vi "Main.vi"() -> ()   [LabVIEW 2017]
doc: "The myRIO Project template acquires acceleration data from the onboard accelerometer and displays the changes of acceleration values in a waveform chart."
uses:
  Motor Status Enum.ctl
  Encoder Cluster.ctl
  <vilib>/myRIO/Common/Instrument Driver Framework/myRIO v1.0/Encoder/typedefs/Encoder Count Direction Enum.ctl
  Motion Type Def.ctl
  XY Cluster.ctl
  <vilib>/myRIO/Instrument Drivers/Onboard IO/PWM/typedefs/PWM Reference.ctl
  <vilib>/myRIO/Common/Instrument Driver Framework/Utilities/typedefs/myRIO Generic Hardware Reference.ctl
  <vilib>/myRIO/Common/Instrument Driver Framework/Utilities/typedefs/Hardware Version Enum.ctl
  <vilib>/myRIO/Common/Instrument Driver Framework/Utilities/typedefs/myRIO v1.0 Reference.ctl
  <vilib>/myRIO/Common/Instrument Driver Framework/Utilities/typedefs/Generic FPGA Reference.ctl
  <vilib>/myRIO/Common/Instrument Driver Framework/myRIO v1.0/PWM/typedefs/PWM Channels Enum.ctl
  <vilib>/myRIO/Instrument Drivers/Onboard IO/PWM/typedefs/PWM Configuration.ctl
  <vilib>/userdefined/High Color/nirio_resource_hc.ctl
  <vilib>/myRIO/Common/Instrument Driver Framework/Utilities/vis/Is FPGA Ref Available.vi
  <vilib>/myRIO/Common/Instrument Driver Framework/myRIO v1.0/PWM/vis/myRIO v1.1 Open PWM.vi
  <vilib>/myRIO/Instrument Drivers/Onboard IO/PWM/vis/Set Duty Cycle and Frequency.vi
  <vilib>/myRIO/Common/Instrument Driver Framework/Utilities/vis/Validate Channels.vi
  <vilib>/myRIO/Common/Instrument Driver Framework/myRIO v1.0/PWM/vis/myRIO v1.0 Reserve PWM.vi
  <vilib>/myRIO/Common/Instrument Driver Framework/myRIO v1.0/UART/vis/myRIO v1.0 Close UART.vi
  <vilib>/myRIO/Common/Instrument Driver Framework/myRIO v1.0/PWM/vis/myRIO v1.0 Build MUX Configuration PWM.vi
  <vilib>/myRIO/Common/Instrument Driver Framework/myRIO v1.0/Resource Manager/vis/myRIO v1.0 Reserve Channel List.vi
  <vilib>/myRIO/Common/Instrument Driver Framework/myRIO v1.0/Resource Manager/vis/myRIO v1.0 Create Configuration List.vi
  <vilib>/myRIO/Common/Instrument Driver Framework/myRIO v1.0/Resource Manager/vis/myRIO v1.0 Reserve Channel.vi
  <vilib>/myRIO/Common/Instrument Driver Framework/myRIO v1.0/Resource Manager/vis/myRIO v1.0 Unreserve Channel.vi
  <vilib>/myRIO/Common/Instrument Driver Framework/myRIO v1.0/Resource Manager/vis/myRIO v1.0 Build Mutex Name.vi
  <vilib>/addons/control/pid/pid.llb/PID Control Input Filter (DBL).vi
  <vilib>/addons/control/pid/pid.llb/PID (DBL).vi
  <vilib>/Utility/VariantDataType/GetNumericInfo.vi
  <vilib>/Utility/error.llb/Error Cluster From Error Code.vi
  <vilib>/myRIO/Common/Instrument Driver Framework/myRIO v1.0/myRIO v1.1 Open.vi
  <vilib>/myRIO/Common/Instrument Driver Framework/Utilities/vis/IO Manager.vi
  <vilib>/myRIO/Common/Instrument Driver Framework/Utilities/vis/Configuration Manager.vi
  <vilib>/myRIO/Common/Instrument Driver Framework/myRIO v1.0/Resource Manager/vis/myRIO v1.0 Configure IO.vi
  <vilib>/myRIO/Common/Instrument Driver Framework/myRIO v1.0/myRIO v1.0 Close.vi
  <vilib>/myRIO/Common/Instrument Driver Framework/myRIO v1.0/PWM/vis/myRIO v1.0 Write PWM.vi
  <vilib>/myRIO/Common/Instrument Driver Framework/Utilities/vis/FPGA Ref Manager.vi
  <vilib>/myRIO/Common/Instrument Driver Framework/myRIO v1.0/myRIO v1.0 Reset FPGA.vi
  <vilib>/myRIO/Common/Instrument Driver Framework/myRIO v1.0/IRQ/vis/myRIO v1.0 IRQ Info FGV.vi
  <vilib>/myRIO/Common/Instrument Driver Framework/myRIO v1.0/IRQ/vis/myRIO v1.0 Timer IRQ Info FGV.vi
  <vilib>/myRIO/Common/Instrument Driver Framework/myRIO v1.0/IRQ/vis/myRIO v1.0 ISR Agent.vi
  <vilib>/myRIO/Express VI/Onboard IO/PWM/PWM Express VI.xnode
  <vilib>/myRIO/Instrument Drivers/Onboard IO/PWM/vis/myRIO PWM Open.xnode
  <vilib>/myRIO/Instrument Drivers/Utilities/Utilities.lvlib
  <vilib>/myRIO/Instrument Drivers/Onboard IO/PWM/PWM.lvlib
  <vilib>/addons/control/pid/NI_PID_pid.lvlib
  <vilib>/ptbypt/NI_PtbyPt.lvlib
panel:
  in  "Y Input":T1
  in  "Y Axis PID":cluster{"Kc":dbl, "Ti":dbl, "Td":dbl}
  in  "X Input":T1
  in  "X Axis PID":cluster{"Kc":dbl, "Ti":dbl, "Td":dbl}
  out "Y dist > +20":bool
  out "X dist > +20":bool
  out "Y Data.Path. Profile":T2=enum."Triangular"
  out "X Data.Path.Profile":T2=enum."Triangular"
  out "Timing":T3
  out "Y PID":cluster{"Speed":dbl, "Speed":dbl}(graph)
  out "X PID":cluster{"Speed":dbl, "Speed":dbl}(graph)
  out "Encoder Output":T4
  out "Y Data.State":T6
  out "X Data.State":T6
  in  "stop":bool
  out "X&Y Complete":bool
  out "Y Displacement":dbl[](graph)
  out "X Displacement":dbl[](graph)
  out "Y Velocity":cluster{"V actual":dbl[]}[](graph)
  out "X Velocity":cluster{"V actual":dbl[]}[](graph)
  out "Y Data.Motion":T7
  out "X Data.Motion":T7
  out "Y Data.Motor Params":T8
  out "X Data.Motor Params":T9
  # "X MaxV = 26.73 mm/s at 50 Hz"
  # "Y MaxV = 14.38 mm/s at 3200 µSteps/rev"
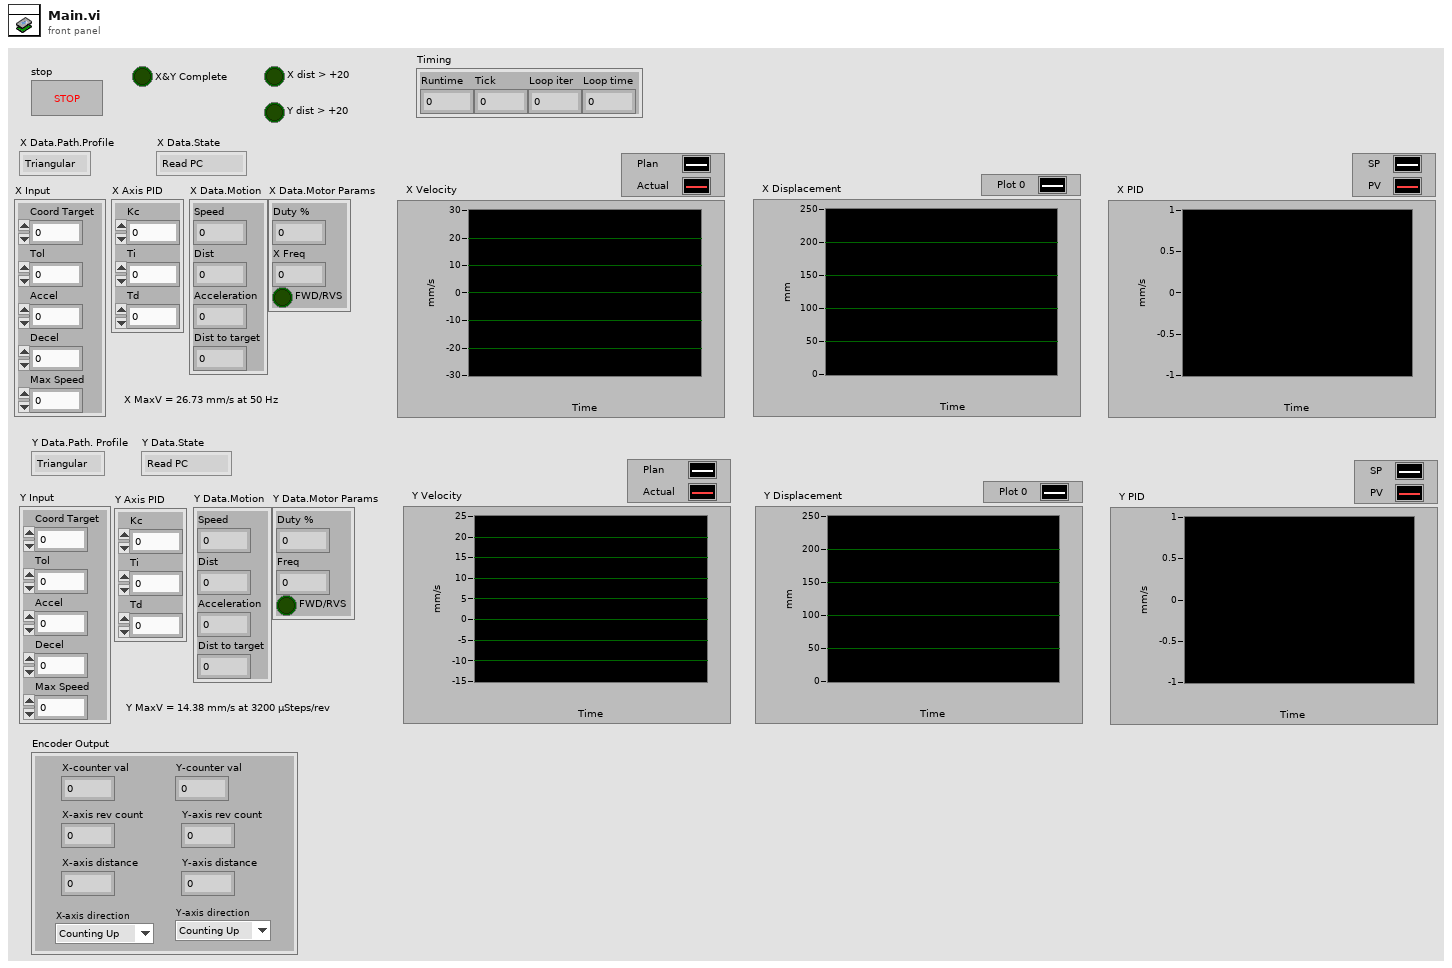
[diagram p1: front panel]
types:
  T1 = cluster{"Coord Target":dbl, "Tol":dbl, "Accel":dbl, "Decel":dbl, "Max Speed":dbl}
  T2 = typedef "Motion Type Def.ctl" = enum16{"Trapezodial", "Triangular"}
  T3 = cluster{"Runtime":dbl, "Loop time":dbl, "Loop iter":i32, "Tick":dbl}
  T4 = typedef "Encoder Cluster.ctl" = cluster{"Y-axis rev count":dbl, "Y-axis distance":dbl, "X-axis rev count":dbl, "X-axis distance":dbl, "Y-axis direction":T5, "X-axis direction":T5, "X-counter val":i32, "Y-counter val":i32}
  T5 = typedef "Encoder Count Direction Enum.ctl" = enum16{"Counting Up", "Counting Down"}
  T6 = typedef "Motor Status Enum.ctl" = enum16{"Read PC", "Stop", "Move"}
  T7 = cluster{"Speed":dbl, "Dist":dbl, "Acceleration":dbl, "Dist to target":dbl}
  T8 = cluster{"Duty %":dbl, "Freq":dbl, "FWD/RVS":bool}
  T9 = cluster{"Duty %":dbl, "X Freq":dbl, "FWD/RVS":bool}
  T10 = typedef "XY Cluster.ctl" = cluster{"X Data":cluster{"Complete?":bool, "Motor Params":cluster{"Duty %":dbl, "X Freq":dbl, "FWD/RVS":bool}, "State":T6, "Input":cluster{"Coord Target":dbl, "Tol":dbl, "Accel":dbl, "Decel":dbl, "Max Speed":dbl}, "Path":cluster{"Speed plan":dbl[], "Profile":T2, "Max Speed":dbl}, "PID":cluster{"Kc":dbl, "Ti":dbl, "Td":dbl}, "Motion":cluster{"Speed":dbl, "Dist":dbl, "Accel":dbl, "Dist Remain":dbl}, "Time step i":i32}, "Y Data":cluster{"Complete?":bool, "Motor Params":cluster{"Duty %":dbl, "Freq":dbl, "FWD/RVS":bool}, "State":T6, "Path":cluster{"Speed plan":dbl[], " Profile":T2, "Max Speed":dbl}, "PID":cluster{"Kc":dbl, "Ti":dbl, "Td":dbl}, "Motion":cluster{"Speed":dbl, "Dist":dbl, "Accel":dbl, "Dist Remain":dbl}, "Input":cluster{"Coord Target":dbl, "Tol":dbl, "Accel":dbl, "Decel":dbl, "Max Speed":dbl}, "Time step i":i32}, "Timing":cluster{"Runtime":dbl, "Loop time":dbl, "Loop iter":i32, "Tick":dbl}, "stop":bool}
  T11 = cluster{"Dist to target (mm)":dbl, "Max Speed (mm/s)":dbl, "Max Accel (mm/s^2)":dbl, "Max Decel (mm/s^2)":dbl, "Step Time (s)":dbl}
  T12 = cluster{"Complete?":bool, "Motor Params":cluster{"Duty %":dbl, "X Freq":dbl, "FWD/RVS":bool}, "State":T6, "Input":cluster{"Coord Target":dbl, "Tol":dbl, "Accel":dbl, "Decel":dbl, "Max Speed":dbl}, "Path":cluster{"Speed plan":dbl[], "Profile":T2, "Max Speed":dbl}, "PID":cluster{"Kc":dbl, "Ti":dbl, "Td":dbl}, "Motion":cluster{"Speed":dbl, "Dist":dbl, "Accel":dbl, "Dist Remain":dbl}, "Time step i":i32}
  T13 = cluster{"Coord Target":bool, "Tol":bool, "Accel":bool, "Decel":bool, "Max Speed":bool}
  T14 = cluster{"Complete?":bool, "Motor Params":cluster{"Duty %":dbl, "Freq":dbl, "FWD/RVS":bool}, "State":T6, "Path":cluster{"Speed plan":dbl[], " Profile":T2, "Max Speed":dbl}, "PID":cluster{"Kc":dbl, "Ti":dbl, "Td":dbl}, "Motion":cluster{"Speed":dbl, "Dist":dbl, "Accel":dbl, "Dist Remain":dbl}, "Input":cluster{"Coord Target":dbl, "Tol":dbl, "Accel":dbl, "Decel":dbl, "Max Speed":dbl}, "Time step i":i32}
  T15 = cluster{"Speed":dbl, "Dist":dbl, "Accel":dbl, "Dist Remain":dbl}
  T16 = cluster{"Runtime":dbl, "Dist":dbl, "Speed":dbl, "Accel":dbl, "Dist":dbl, "Speed":dbl, "Accel":dbl}
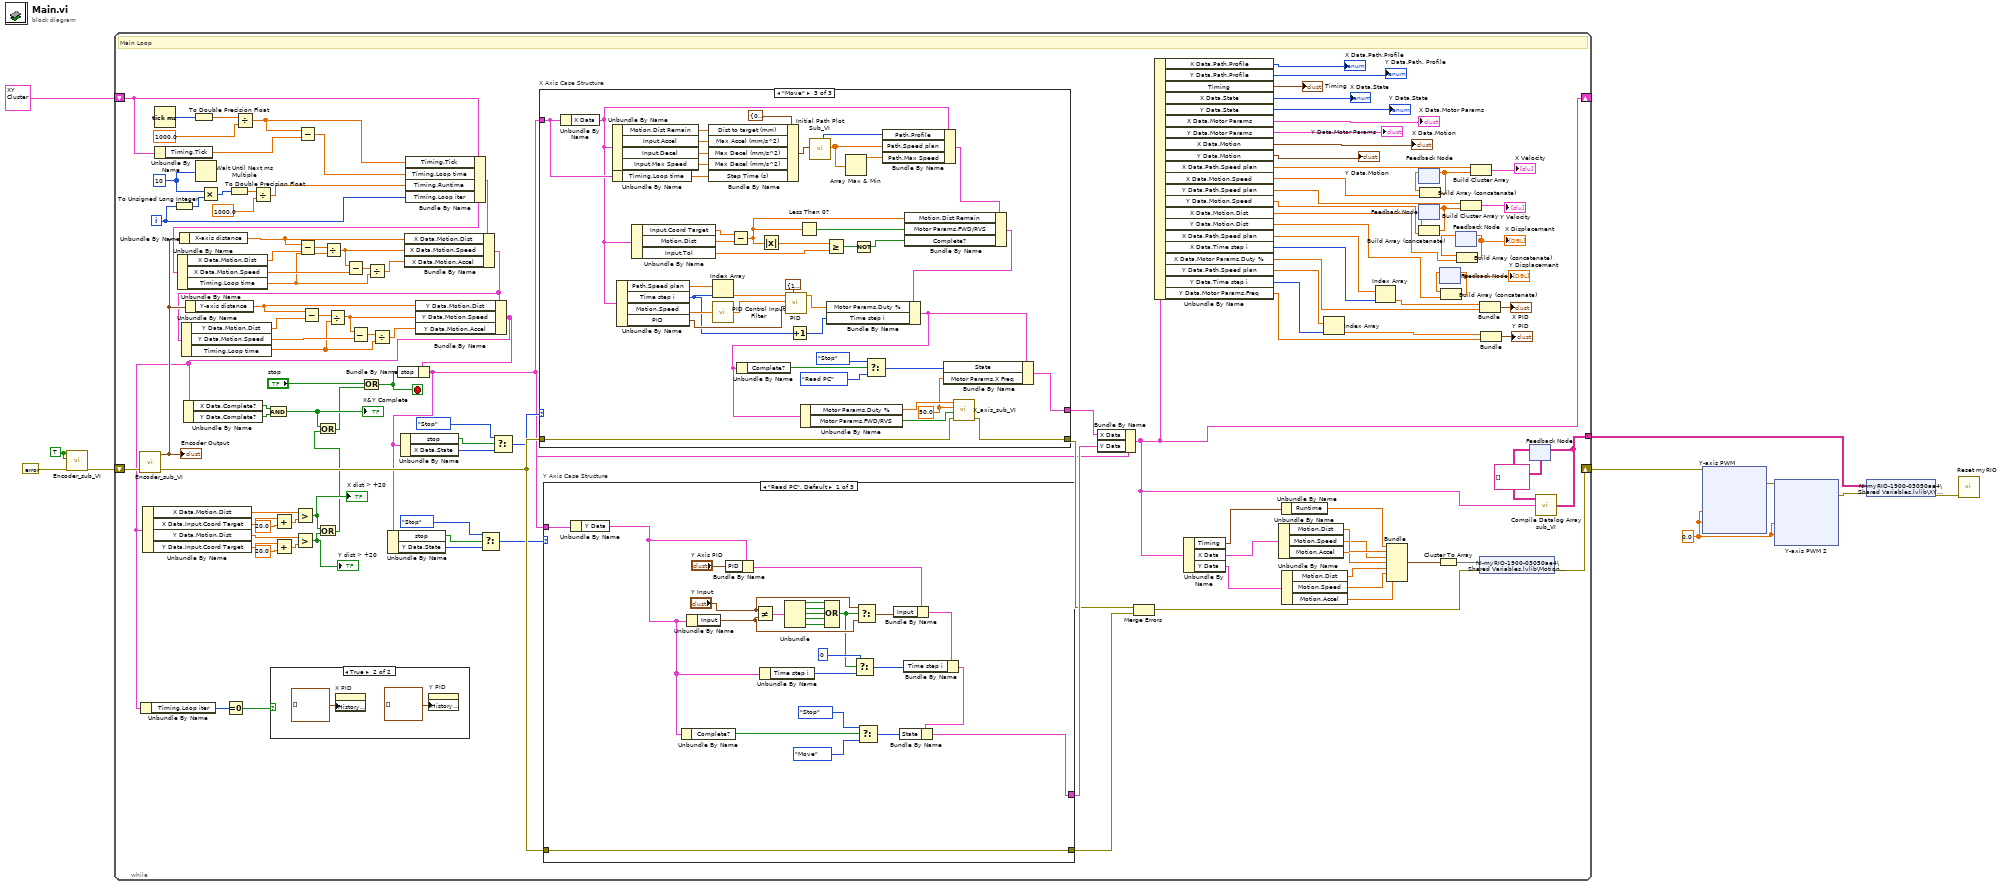
[diagram p0: block diagram]
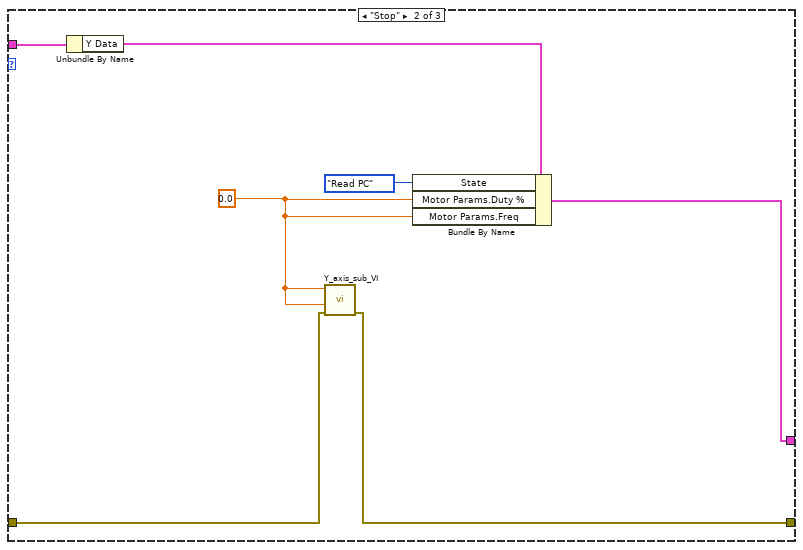
[diagram p3: hidden frame]
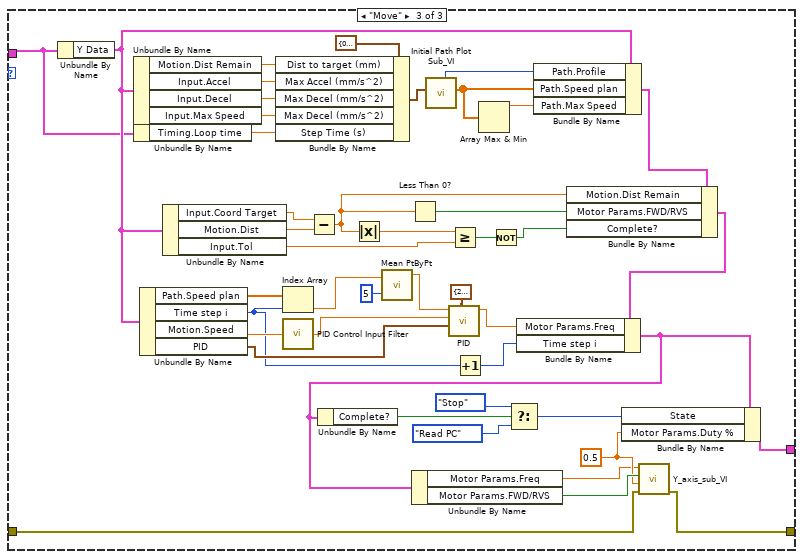
[diagram p4: hidden frame]
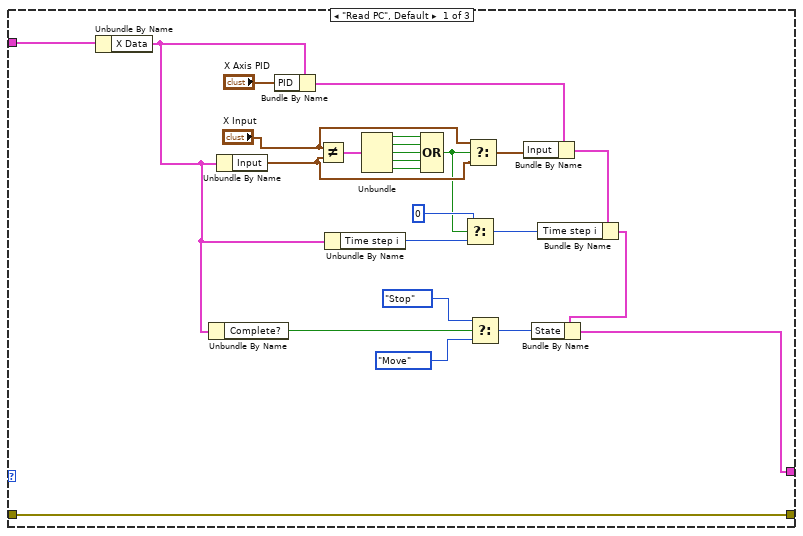
[diagram p5: hidden frame]
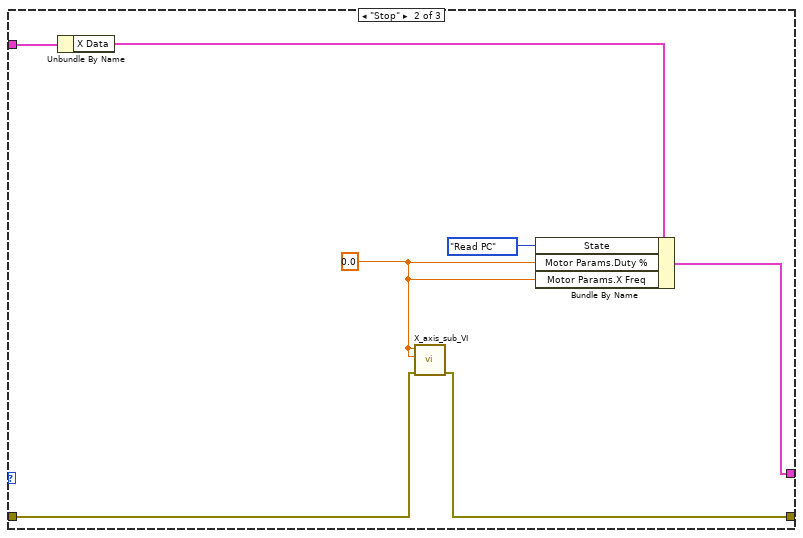
[diagram p6: hidden frame]
diagram:
  w4 = TRUE ("Reset X Counter")
  w9 = 0.0 ("Frequency [Hz]")
  n1 = call "Encoder_sub_VI.vi"("error in (no error)"=errorcluster {"status"=FALSE, "code"=0, "source"=""}, "Reset Y Counter"=w4, "Reset X Counter"=w4) -> ("error out"=w5:errorcluster)  [unwired: 7 in, 1 out]
  n2 = while {
    shift-right: [w45] -> w7
    shift-left: w5 -> [w131]
    shift-right: [w44] -> _
    shift-left: T10 {"X Data"={"Complete?"=FALSE, "Motor Params"={"Duty %"=0.0, "X Freq"=0.0, "FWD/RVS"=FALSE}, "State"=enum."Read PC", "Input"={"Coord Target"=0.0, "Tol"=0.0, "Accel"=0.0, "Decel"=0.0, "Max Speed"=0.0}, "Path"={"Speed plan"=[], "Profile"=enum."Triangular", "Max Speed"=0.0}, "PID"={"Kc"=0.0, "Ti"=0.0, "Td"=0.0}, "Motion"={"Speed"=0.0, "Dist"=0.0, "Accel"=0.0, "Dist Remain"=0.0}, "Time step i"=0}, "Y Data"={"Complete?"=FALSE, "Motor Params"={"Duty %"=0.0, "Freq"=0.0, "FWD/RVS"=FALSE}, "State"=enum."Read PC", "Path"={"Speed plan"=[], " Profile"=enum."Triangular", "Max Speed"=0.0}, "PID"={"Kc"=0.0, "Ti"=0.0, "Td"=0.0}, "Motion"={"Speed"=0.0, "Dist"=0.0, "Accel"=0.0, "Dist Remain"=0.0}, "Input"={"Coord Target"=0.0, "Tol"=0.0, "Accel"=0.0, "Decel"=0.0, "Max Speed"=0.0}, "Time step i"=0}, "Timing"={"Runtime"=0.0, "Loop time"=0.0, "Loop iter"=0, "Tick"=0.0}, "stop"=FALSE} ("XY Cluster 2") -> [w85]
    tunnel: [w99] -> w3
    i -> [w125]
    stop <- w61 stop-if-true
    w124 = u32 10 ("millisecond multiple")
    # "Main Loop"
    n3 = call "Encoder_sub_VI.vi"("error in (no error)"=w131) -> ("error out"=w103:errorcluster, "Encoder Output"=w112:T4)  [unwired: 9 in]
    "Encoder Output" <- w112
    n4 = Tick Count (ms)() -> (millisecond timer value=w118:u32)
    n5 = Unbundle By Name(w85) -> ("Timing.Tick"=w84:dbl)
    n6 = To Unsigned Long Integer(number=w125) -> (unsigned 32bit integer=w123:u32)
    n7 = Unbundle By Name(w112) -> ("X-axis distance"=w129:dbl)
    n8 = Unbundle By Name(w112) -> ("Y-axis distance"=w104:dbl)
    n9 = To Double Precision Float(number=w118) -> (double precision float=w86:dbl)
    n10 = Wait Until Next ms Multiple(millisecond multiple=w124) -> ()  [unwired: 1 out]
    n11 = Multiply(x=w124, y=w123) -> (x*y=w122:u32)
    n12 = To Double Precision Float(number=w122) -> (double precision float=w120:dbl)
    n13 = Divide(x=w86, y=1000.0) -> (x/y=w83:dbl)
    n14 = Divide(x=w120, y=1000.0) -> (x/y=w119:dbl)
    n15 = Subtract(x=w83, y=w84) -> (x-y=w82:dbl)
    n16 = Bundle By Name(cluster=w85, "Timing.Tick"=w83, "Timing.Loop time"=w82, "Timing.Runtime"=w119, "Timing.Loop iter"=w125) -> (w126:T10)
    n17 = Unbundle By Name(w126) -> ("X Data.Motion.Dist"=w128:dbl, "X Data.Motion.Speed"=w115:dbl, "Timing.Loop time"=w113:dbl)
    n18 = Subtract(x=w129, y=w128) -> (x-y=w127:dbl)
    n19 = Divide(x=w127, y=w113) -> (x/y=w114:dbl)
    n20 = Subtract(x=w114, y=w115) -> (x-y=w116:dbl)
    n21 = Divide(x=w116, y=w113) -> (x/y=w60:dbl)
    n22 = Bundle By Name(cluster=w126, "X Data.Motion.Dist"=w129, "X Data.Motion.Speed"=w114, "X Data.Motion.Accel"=w60) -> (w105:T10)
    n23 = Unbundle By Name(w105) -> ("Y Data.Motion.Dist"=w111:dbl, "Y Data.Motion.Speed"=w108:dbl, "Timing.Loop time"=w106:dbl)
    n24 = Subtract(x=w104, y=w111) -> (x-y=w110:dbl)
    n25 = Divide(x=w110, y=w106) -> (x/y=w107:dbl)
    n26 = Subtract(x=w107, y=w108) -> (x-y=w109:dbl)
    n27 = Divide(x=w109, y=w106) -> (x/y=w59:dbl)
    n28 = Bundle By Name(cluster=w105, "Y Data.Motion.Dist"=w104, "Y Data.Motion.Speed"=w107, "Y Data.Motion.Accel"=w59) -> (w66:T10)
    n29 = Unbundle By Name(w66) -> ("Timing.Loop iter"=w64:i32)
    n30 = Unbundle By Name(w66) -> ("X Data.Motion.Dist"=w78:dbl, "X Data.Input.Coord Target"=w71:dbl, "Y Data.Motion.Dist"=w76:dbl, "Y Data.Input.Coord Target"=w68:dbl)
    n31 = Unbundle By Name(w66) -> ("X Data.Complete?"=w88:bool, "Y Data.Complete?"=w87:bool)
    n32 = Equal To 0?(x=w64) -> (x = 0?=w65:bool)
    n33 = And(x=w88, y=w87) -> (x .and. y?=w74:bool)
    "X&Y Complete" <- w74
    n34 = case shown="True" w65 {
      frame False {
      }
      frame True {
        n35 = property on="X PID" class="WFChart (strict)"("History Data"=cluster{"Speed":dbl, "Speed":dbl}[] []) -> ()  [unwired: 2 in, 2 out]
        n36 = property on="Y PID" class="WFChart (strict)"("History Data"=cluster{"Speed":dbl, "Speed":dbl}[] []) -> ()  [unwired: 2 in, 2 out]
      }
    }
    n37 = Add(x=w71, y=20.0) -> (x+y=w70:dbl)
    n38 = Add(x=w68, y=20.0) -> (x+y=w67:dbl)
    n39 = Greater?(x=w78, y=w70) -> (0:w77:bool)
    "X dist > +20" <- w77
    n40 = Greater?(x=w76, y=w67) -> (0:w73:bool)
    "Y dist > +20" <- w73
    n41 = Or(x=w77, y=w73) -> (x .or. y?=w75:bool)
    n42 = Or(x=w74, y=w75) -> (x .or. y?=w62:bool)
    n43 = Or(x="stop", y=w62) -> (x .or. y?=w61:bool)
    n44 = Bundle By Name(cluster=w66, "stop"=w61) -> (w81:T10)
    n45 = Unbundle By Name(w81) -> ("stop"=w91:bool, "Y Data.State"=w92:T6)
    n46 = Unbundle By Name(w81) -> ("stop"=w95:bool, "X Data.State"=w96:T6)
    n47 = Select(t=Motor_Status_Enum."Stop", s=w91, f=w92) -> (s? t:f=w89:T6)
    n48 = Select(t=Motor_Status_Enum."Stop", s=w95, f=w96) -> (s? t:f=w93:T6)
    n49 = case "X Axis Case Structure" shown="\"Move\"" w93 {
      tunnel: [w213 w241 w250] -> w130
      tunnel: w103 -> [w233 w238 w246]
      tunnel: [w233 w237 w245] -> w101
      tunnel: w81 -> [w234 w240 w274]
      frame "Read PC", Default {
        n50 = Unbundle By Name(w234) -> ("X Data"=w211:T12)
        n51 = Unbundle By Name(w211) -> ("Complete?"=w210:bool)
        n52 = Unbundle By Name(w211) -> ("Input"=w223:T1)
        n53 = Bundle By Name(cluster=w211, "PID"="X Axis PID") -> (w231:T12)
        n54 = Not Equal?(x="X Input", y=w223) -> (x != y?=w230:T13)
        n55 = Unbundle By Name(w211) -> ("Time step i"=w212:i32)
        n56 = Unbundle(w230) -> ("Coord Target"=w229:bool, "Tol"=w228:bool, "Accel"=w227:bool, "Decel"=w226:bool, "Max Speed"=w225:bool)
        n57 = Compound Arithmetic op=OR(w229, w228, w227, w226, w225) -> (w215:bool)
        n58 = Select(t=0 ("Motor Params.Duty %"), s=w215, f=w212) -> (s? t:f=w220:i32)
        n59 = Select(t="X Input", s=w215, f=w223) -> (s? t:f=w222:T1)
        n60 = Select(t=Motor_Status_Enum."Stop" ("State"), s=w210, f=Motor_Status_Enum."Move" ("State")) -> (s? t:f=w218:T6)
        n61 = Bundle By Name(cluster=w231, "Input"=w222) -> (w219:T12)
        n62 = Bundle By Name(cluster=w219, "Time step i"=w220) -> (w214:T12)
        n63 = Bundle By Name(cluster=w214, "State"=w218) -> (w213:T12)
      }
      frame "Stop" {
        w235 = 0.0 ("Frequency")
        n64 = Unbundle By Name(w240) -> ("X Data"=w239:T12)
        n65 = call "X_axis_sub_VI.vi"("error in (no error)"=w238, "Frequency"=w235, "Duty Cycle %"=w235) -> ("error out"=w237:errorcluster)  [unwired: 8 in]
        n66 = Bundle By Name(cluster=w239, "State"=Motor_Status_Enum."Read PC", "Motor Params.Duty %"=w235, "Motor Params.X Freq"=w235) -> (w241:T12)
      }
      frame "Move" {
        w242 = 50.0 ("Frequency")
        n67 = Unbundle By Name(w274) -> ("X Data"=w248:T12)
        n68 = Unbundle By Name(w248) -> ("Motion.Dist Remain"=w267:dbl, "Input.Accel"=w266:dbl, "Input.Decel"=w265:dbl, "Input.Max Speed"=w264:dbl)
        n69 = Unbundle By Name(w274) -> ("Timing.Loop time"=w273:dbl)
        n70 = Unbundle By Name(w248) -> ("Path.Speed plan"=w254:dbl[], "Time step i"=w252:i32, "Motion.Speed"=w259:dbl, "PID"=w258:cluster{"Kc":dbl, "Ti":dbl, "Td":dbl})
        n71 = Unbundle By Name(w248) -> ("Input.Coord Target"=w271:dbl, "Motion.Dist"=w280:dbl, "Input.Tol"=w283:dbl)
        n72 = Bundle By Name(cluster=T11 {"Dist to target (mm)"=0.0, "Max Speed (mm/s)"=0.0, "Max Accel (mm/s^2)"=0.0, "Max Decel (mm/s^2)"=0.0, "Step Time (s)"=0.0} ("Motion Inputs"), "Dist to target (mm)"=w267, "Max Accel (mm/s^2)"=w266, "Max Decel (mm/s^2)"=w265, "Max Decel (mm/s^2)"=w264, "Step Time (s)"=w273) -> (w276:T11)
        n73 = Index Array(array=w254, index=w252) -> (element=w253:dbl)
        n74 = call-poly <vilib>:"PID Control Input Filter.vi"("input"=w259) -> ("output"=w260:dbl)  [unwired: 4 in]
        n75 = Subtract(x=w271, y=w280) -> (x-y=w270:dbl)
        n76 = Absolute Value(x=w270) -> (abs(x)=w268:dbl)
        n77 = call-poly <vilib>:"PID.vi"("output range"=cluster{"output high":dbl, "output low":dbl} {"output high"=100.0, "output low"=0.0}, "PID gains"=w258, "process variable"=w260, "setpoint"=w253) -> ("output"=w256:dbl)  [unwired: 6 in, 1 out]
        n78 = Increment(x=w252) -> (x+1=w251:i32)
        n79 = Less Than 0?(x=w270) -> (x < 0?=w269:bool)
        n80 = call "Initial Path Plot Sub_VI.vi"("Motion Inputs"=w276) -> ("Velocity Array"=w262:dbl[], "Motion Profile"=w272:T2)  [unwired: 6 in, 3 out]
        n81 = Greater Or Equal?(x=w268, y=w283) -> (x >= y?=w282:bool)
        n82 = Array Max & Min(array=w262) -> (max value=w263:dbl)  [unwired: 3 out]
        n83 = Not(x=w282) -> (.not. x?=w281:bool)
        n84 = Bundle By Name(cluster=w248, "Path.Profile"=w272, "Path.Speed plan"=w262, "Path.Max Speed"=w263) -> (w261:T12)
        n85 = Bundle By Name(cluster=w261, "Motion.Dist Remain"=w270, "Motor Params.FWD/RVS"=w269, "Complete?"=w281) -> (w257:T12)
        n86 = Bundle By Name(cluster=w257, "Motor Params.Duty %"=w256, "Time step i"=w251) -> (w244:T12)
        n87 = Unbundle By Name(w244) -> ("Complete?"=w249:bool)
        n88 = Unbundle By Name(w244) -> ("Motor Params.Duty %"=w243:dbl, "Motor Params.FWD/RVS"=w247:bool)
        n89 = Select(t=Motor_Status_Enum."Stop" ("State"), s=w249, f=Motor_Status_Enum."Read PC" ("State")) -> (s? t:f=w278:T6)
        n90 = Bundle By Name(cluster=w244, "State"=w278, "Motor Params.X Freq"=w242) -> (w250:T12)
        n91 = call "X_axis_sub_VI.vi"("error in (no error)"=w246, "FWD/RVS"=w247, "Frequency"=w242, "Duty Cycle %"=w243) -> ("error out"=w245:errorcluster)  [unwired: 7 in]
      }
    }
    n92 = case "Y Axis Case Structure" shown="\"Read PC\", Default" w89 {
      tunnel: [w134 w161 w173] -> w102
      tunnel: w103 -> [w157 w160 w170]
      tunnel: [w157 w159 w169] -> w100
      tunnel: w81 -> [w158 w165 w174]
      frame "Read PC", Default {
        n93 = Unbundle By Name(w158) -> ("Y Data"=w135:T14)
        n94 = Unbundle By Name(w135) -> ("Complete?"=w136:bool)
        n95 = Unbundle By Name(w135) -> ("Input"=w147:T1)
        n96 = Bundle By Name(cluster=w135, "PID"="Y Axis PID") -> (w155:T14)
        n97 = Not Equal?(x="Y Input", y=w147) -> (x != y?=w154:T13)
        n98 = Unbundle By Name(w135) -> ("Time step i"=w137:i32)
        n99 = Unbundle(w154) -> ("Coord Target"=w153:bool, "Tol"=w152:bool, "Accel"=w151:bool, "Decel"=w150:bool, "Max Speed"=w149:bool)
        n100 = Compound Arithmetic op=OR(w153, w152, w151, w150, w149) -> (w139:bool)
        n101 = Select(t=0 ("Motor Params.Duty %"), s=w139, f=w137) -> (s? t:f=w144:i32)
        n102 = Select(t="Y Input", s=w139, f=w147) -> (s? t:f=w146:T1)
        n103 = Select(t=Motor_Status_Enum."Stop" ("State"), s=w136, f=Motor_Status_Enum."Move" ("State")) -> (s? t:f=w142:T6)
        n104 = Bundle By Name(cluster=w155, "Input"=w146) -> (w143:T14)
        n105 = Bundle By Name(cluster=w143, "Time step i"=w144) -> (w138:T14)
        n106 = Bundle By Name(cluster=w138, "State"=w142) -> (w134:T14)
      }
      frame "Stop" {
        w163 = 0.0 ("Frequency")
        n107 = Unbundle By Name(w165) -> ("Y Data"=w162:T14)
        n108 = call "Y_axis_sub_VI.vi"("error in (no error)"=w160, "Duty Cycle"=w163, "Frequency"=w163) -> ("error out"=w159:errorcluster)  [unwired: 8 in]
        n109 = Bundle By Name(cluster=w162, "State"=Motor_Status_Enum."Read PC", "Motor Params.Duty %"=w163, "Motor Params.Freq"=w163) -> (w161:T14)
      }
      frame "Move" {
        w172 = 0.5 ("Frequency")
        n110 = Unbundle By Name(w174) -> ("Y Data"=w177:T14)
        n111 = Unbundle By Name(w177) -> ("Motion.Dist Remain"=w194:dbl, "Input.Accel"=w193:dbl, "Input.Decel"=w192:dbl, "Input.Max Speed"=w191:dbl)
        n112 = Unbundle By Name(w174) -> ("Timing.Loop time"=w200:dbl)
        n113 = Unbundle By Name(w177) -> ("Path.Speed plan"=w181:dbl[], "Time step i"=w180:i32, "Motion.Speed"=w186:dbl, "PID"=w185:cluster{"Kc":dbl, "Ti":dbl, "Td":dbl})
        n114 = Unbundle By Name(w177) -> ("Input.Coord Target"=w198:dbl, "Motion.Dist"=w206:dbl, "Input.Tol"=w209:dbl)
        n115 = Bundle By Name(cluster=T11 {"Dist to target (mm)"=0.0, "Max Speed (mm/s)"=0.0, "Max Accel (mm/s^2)"=0.0, "Max Decel (mm/s^2)"=0.0, "Step Time (s)"=0.0} ("Motion Inputs"), "Dist to target (mm)"=w194, "Max Accel (mm/s^2)"=w193, "Max Decel (mm/s^2)"=w192, "Max Decel (mm/s^2)"=w191, "Step Time (s)"=w200) -> (w202:T11)
        n116 = Index Array(array=w181, index=w180) -> (element=w167:dbl)
        n117 = call-poly <vilib>:"PID Control Input Filter.vi"("input"=w186) -> ("output"=w187:dbl)  [unwired: 4 in]
        n118 = Subtract(x=w198, y=w206) -> (x-y=w197:dbl)
        n119 = Absolute Value(x=w197) -> (abs(x)=w195:dbl)
        n120 = call <vilib>:"Mean PtByPt.vi"("x"=w167, "sample length"=5) -> ("mean"=w168:dbl)  [unwired: 2 in, 1 out]
        n121 = Less Than 0?(x=w197) -> (x < 0?=w196:bool)
        n122 = call "Initial Path Plot Sub_VI.vi"("Motion Inputs"=w202) -> ("Velocity Array"=w189:dbl[], "Motion Profile"=w199:T2)  [unwired: 6 in, 3 out]
        n123 = call-poly <vilib>:"PID.vi"("output range"=cluster{"output high":dbl, "output low":dbl} {"output high"=23000.0, "output low"=0.0}, "PID gains"=w185, "process variable"=w187, "setpoint"=w168) -> ("output"=w183:dbl)  [unwired: 6 in, 1 out]
        n124 = Greater Or Equal?(x=w195, y=w209) -> (x >= y?=w208:bool)
        n125 = Increment(x=w180) -> (x+1=w179:i32)
        n126 = Array Max & Min(array=w189) -> (max value=w190:dbl)  [unwired: 3 out]
        n127 = Not(x=w208) -> (.not. x?=w207:bool)
        n128 = Bundle By Name(cluster=w177, "Path.Profile"=w199, "Path.Speed plan"=w189, "Path.Max Speed"=w190) -> (w188:T14)
        n129 = Bundle By Name(cluster=w188, "Motion.Dist Remain"=w197, "Motor Params.FWD/RVS"=w196, "Complete?"=w207) -> (w184:T14)
        n130 = Bundle By Name(cluster=w184, "Motor Params.Freq"=w183, "Time step i"=w179) -> (w175:T14)
        n131 = Unbundle By Name(w175) -> ("Complete?"=w178:bool)
        n132 = Unbundle By Name(w175) -> ("Motor Params.Freq"=w171:dbl, "Motor Params.FWD/RVS"=w176:bool)
        n133 = Select(t=Motor_Status_Enum."Stop" ("State"), s=w178, f=Motor_Status_Enum."Read PC" ("State")) -> (s? t:f=w204:T6)
        n134 = Bundle By Name(cluster=w175, "State"=w204, "Motor Params.Duty %"=w172) -> (w173:T14)
        n135 = call "Y_axis_sub_VI.vi"("error in (no error)"=w170, "Duty Cycle"=w172, "FWD/RVS"=w176, "Frequency"=w171) -> ("error out"=w169:errorcluster)  [unwired: 7 in]
      }
    }
    n136 = Bundle By Name(cluster=w81, "X Data"=w130, "Y Data"=w102) -> (w44:T10)
    n137 = Merge Errors(w101, w100) -> (w46:errorcluster)
    n138 = Unbundle By Name(w44) -> ("X Data.Path.Profile"=→"X Data.Path.Profile":T2, "Y Data.Path.Profile"=→"Y Data.Path. Profile":T2, "Timing"=→"Timing":T3, "X Data.State"=→"X Data.State":T6, "Y Data.State"=→"Y Data.State":T6, "X Data.Motor Params"=→"X Data.Motor Params":T9, "Y Data.Motor Params"=→"Y Data.Motor Params":T8, "X Data.Motion"=→"X Data.Motion":T15, "Y Data.Motion"=→"Y Data.Motion":T15, "X Data.Path.Speed plan"=w80:dbl[], "X Data.Motion.Speed"=w32:dbl, "Y Data.Path.Speed plan"=w79:dbl[], "Y Data.Motion.Speed"=w29:dbl, "X Data.Motion.Dist"=w25:dbl, "Y Data.Motion.Dist"=w23:dbl, "X Data.Path.Speed plan"=w18:dbl[], "X Data.Time step i"=w17:i32, "X Data.Motor Params.Duty %"=w20:dbl, "Y Data.Path.Speed plan"=w14:dbl[], "Y Data.Time step i"=w13:i32, "Y Data.Motor Params.Freq"=w15:dbl)
    n139 = Unbundle By Name(w44) -> ("Timing"=w48:T3, "X Data"=w58:T12, "Y Data"=w57:T14)
    n140 = Unbundle By Name(w58) -> ("Motion.Dist"=w56:dbl, "Motion.Speed"=w55:dbl, "Motion.Accel"=w54:dbl)
    n141 = Unbundle By Name(w48) -> ("Runtime"=w47:dbl)
    n142 = Unbundle By Name(w57) -> ("Motion.Dist"=w53:dbl, "Motion.Speed"=w52:dbl, "Motion.Accel"=w51:dbl)
    n143 = Index Array(array=w14, index=w13) -> (element=w12:dbl)
    n144 = Index Array(array=w18, index=w17) -> (element=w16:dbl)
    n145 = Bundle("Runtime"=w47, "Dist"=w56, "Speed"=w55, "Accel"=w54, "Dist"=w53, "Speed"=w52, "Accel"=w51) -> (w50:T16)  [unwired: 1 in]
    n146 = feedback #1() -> (w27:dbl[])  [unwired: 1 in]
    n147 = feedback #2() -> (w31:dbl[])  [unwired: 1 in]
    n148 = Build Array (concatenate)(w27, w29) -> (w28:dbl[])
    n149 = feedback-in #1(w28) -> ()
    n150 = Build Array (concatenate)(w31, w32) -> (w30:dbl[])
    n151 = feedback-in #2(w30) -> ()
    n152 = Cluster To Array(cluster=w50) -> (array=w49:dbl[])
    n153 = feedback #3() -> (w22:dbl[])  [unwired: 1 in]
    n154 = Build Array (concatenate)(w22, w23) -> (w21:dbl[])
    "Y Displacement" <- w21
    n155 = feedback-in #3(w21) -> ()
    n156 = feedback #4() -> (w24:dbl[])  [unwired: 1 in]
    n157 = Build Array (concatenate)(w24, w25) -> (w26:dbl[])
    "X Displacement" <- w26
    n158 = feedback-in #4(w26) -> ()
    n159 = Build Cluster Array(w79, w28) -> (→"Y Velocity":cluster{"Speed plan":dbl[]}[])
    n160 = Build Cluster Array(w80, w30) -> (→"X Velocity":cluster{"Speed plan":dbl[]}[])
    n161 = Bundle("Numeric"=w16, "Duty %"=w20) -> (→"X PID":cluster{"Numeric":dbl, "Duty %":dbl})  [unwired: 1 in]
    n162 = shared-variable "NI-myRIO-1900-03050ae4\\Shared Variables.lvlib\\Motion Data"(w49, error in=w46) -> (error out=w45:errorcluster)
    n163 = Bundle("Numeric"=w12, "Freq"=w15) -> (→"Y PID":cluster{"Numeric":dbl, "Freq":dbl})  [unwired: 1 in]
    n164 = feedback #5(string[][] [] ("Initialised Array")) -> (w98:string[][])
    n165 = call "Compile Datalog Array sub_VI.vi"("XY Cluster"=w44, "Initialised Array"=w98) -> ("Data Array"=w99:string[][])  [unwired: 1 in]
    n166 = feedback-in #5(w99) -> ()
  }
  n167 = xnode "Y-axis PWM"("Duty Cycle"=w9, "Frequency [Hz]"=w9, "error in (no error)"=w7) -> ("error out"=w10:errorcluster)
  n168 = xnode "Y-axis PWM 2"("Duty Cycle"=w9, "Frequency [Hz]"=w9, "error in (no error)"=w10) -> ("error out"=w1:errorcluster)
  n169 = shared-variable "NI-myRIO-1900-03050ae4\\Shared Variables.lvlib\\XY Datalog"(w3, error in=w1) -> (error out=w2:errorcluster)
  n170 = call <vilib>:"Reset myRIO.vi"("error in (no error)"=w2) -> ()  [unwired: 10 in, 1 out]
